vi "GetData.vi"(8 "error in (no error)":errorcluster, 10 "DATA":string(combo)="ATDATA", 11 "VISA Refnum in":refnum<visa-resource-name>) -> (0 "error out":errorcluster, 2 "data":string, 3 "VISA Refnum out":refnum<visa-resource-name>)   [LabVIEW 2011]
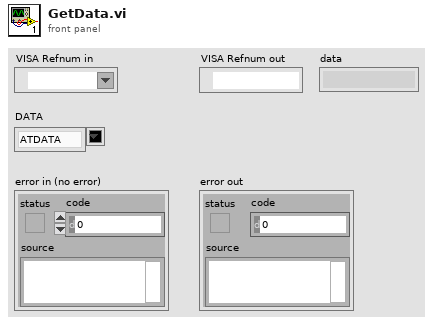
[diagram p1: front panel]
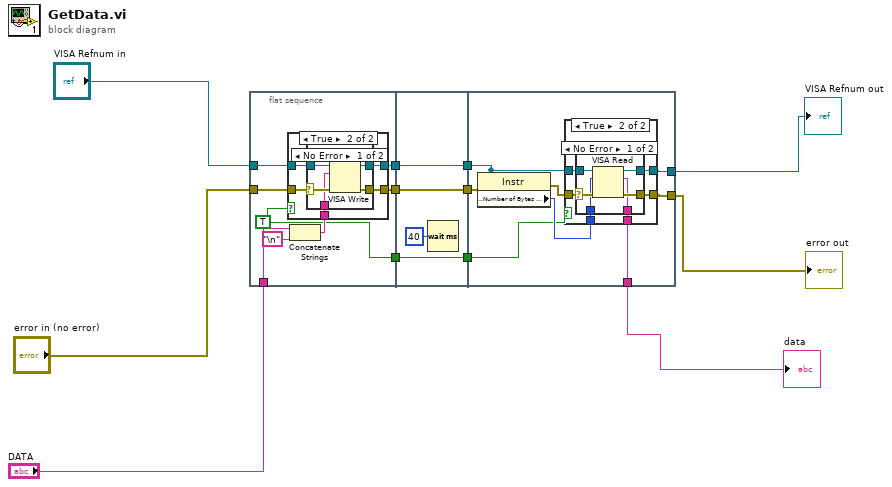
[diagram p0: block diagram]
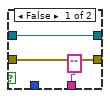
[diagram p4: hidden frame]
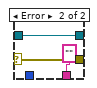
[diagram p5: hidden frame]
diagram:
  n1 = flat-sequence {
    tunnel: [w18] -> w12
    tunnel: [w17] -> w11
    tunnel: "VISA Refnum in" -> [w16]
    tunnel: [w15] -> w10
    tunnel: "error in (no error)" -> [w14]
    tunnel: "DATA" -> [w13]
    tunnel: [w37] -> w9
    tunnel: w12 -> [w37]
    tunnel: w11 -> [w36]
    tunnel: [w36] -> w8
    tunnel: [w35] -> w7
    tunnel: w10 -> [w35]
    tunnel: w9 -> [w44]
    tunnel: w8 -> [w43]
    tunnel: w7 -> [w42]
    tunnel: [w39] -> w1
    tunnel: [w41] -> w2
    tunnel: [w40] -> w5
    frame #0 {
      w15 = TRUE
      n2 = Concatenate Strings(w13, "\n") -> (w19:string)
      n3 = case shown="True" w15 {
        tunnel: [w22 w27] -> w18
        tunnel: [w21 w26] -> w17
        tunnel: w16 -> [w22 w25]
        tunnel: w14 -> [w21 w24]
        tunnel: w19 -> [_ w23]
        frame False {
        }
        frame True {
          n4 = case shown="No Error" w24 {
            selector: w24 -> [w29 w34]
            tunnel: [w32 w33] -> w27
            tunnel: [w31 w34] -> w26
            tunnel: w25 -> [w30 w33]
            tunnel: w23 -> [w28 _]
            frame No Error {
              n5 = VISA Write(VISA resource name=w30, write buffer=w28, error in (no error)=w29) -> (VISA resource name out=w32:refnum<visa-resource-name>, error out=w31:errorcluster)  [unwired: 1 out]
            }
            frame Error {
            }
          }
        }
      }
    }
    frame #1 {
      n6 = Wait (ms)(milliseconds to wait=u32 40) -> ()  [unwired: 1 out]
    }
    frame #2 {
      n7 = property class="Instr"(reference=w44, error in=w43) -> (error out=w46:errorcluster, "Serial Settings:Number of Bytes at Serial Port"=w45:u32)  [unwired: 1 out]
      n8 = case shown="True" w42 {
        tunnel: [w49 w55] -> w39
        tunnel: [w48 w54] -> w41
        tunnel: w44 -> [w49 w53]
        tunnel: w46 -> [w48 w52]
        tunnel: ["" ("read buffer") w51] -> w40
        tunnel: w45 -> [_ w50]
        frame False {
        }
        frame True {
          n9 = case shown="No Error" w52 {
            selector: w52 -> [w58 w64]
            tunnel: [w61 w63] -> w55
            tunnel: [w60 w64] -> w54
            tunnel: w53 -> [w59 w63]
            tunnel: [w57 "" ("read buffer")] -> w51
            tunnel: w50 -> [w56 _]
            frame No Error {
              n10 = VISA Read(VISA resource name=w59, byte count=w56, error in (no error)=w58) -> (VISA resource name out=w61:refnum<visa-resource-name>, read buffer=w57:string, error out=w60:errorcluster)  [unwired: 1 out]
            }
            frame Error {
            }
          }
        }
      }
    }
  }
  "VISA Refnum out" <- w1
  "error out" <- w2
  "data" <- w5
